vi "INI Configs FGV.vi"(6 "Config File Path":path, 7 "State":T1, 8 "error in":errorcluster, 9 "key":string, 10 "value in":string, 11 "section":string) -> (0 "error out":errorcluster, 3 "value":string)   [LabVIEW 2021]
doc: "This FGV is used to read/write config files which would contain the general configs of the application. \nBasic \"String\" config read write is implemented but it can be extended to cater to all data types."
uses:
  controls/INI FGV States.ctl
  <vilib>/Utility/config.llb/Read Key (String).vi
  <vilib>/Utility/config.llb/Write Key (String).vi
  <vilib>/Utility/config.llb/NI_LVConfig.lvlib
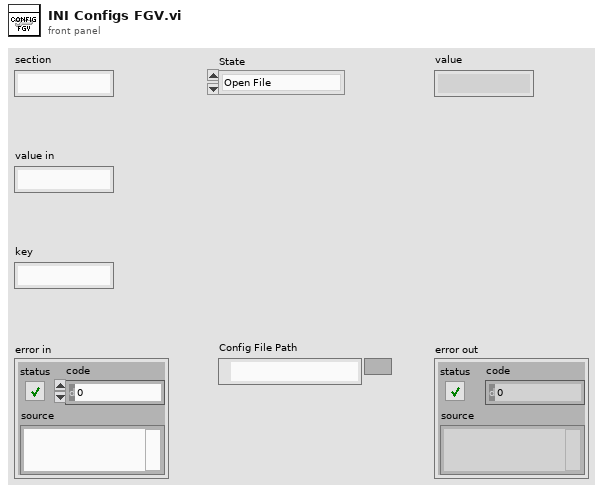
[diagram p1: front panel]
types:
  T1 = typedef "INI FGV States.ctl" = enum16{"Open File", "Read Config", "Write Config", "Close File"}
  T2 = typedef "NI_LVConfig.lvlib/Config Data RefNum.ctl" = refnum<k1>
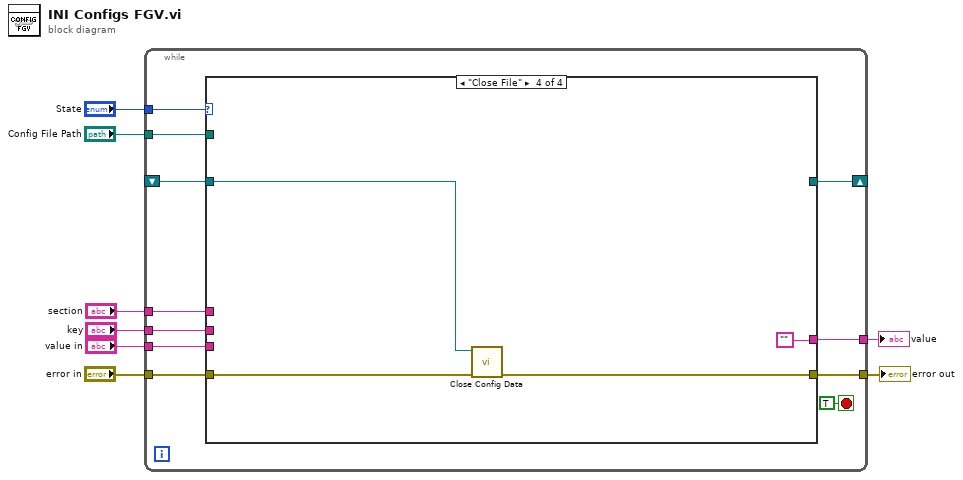
[diagram p0: block diagram]
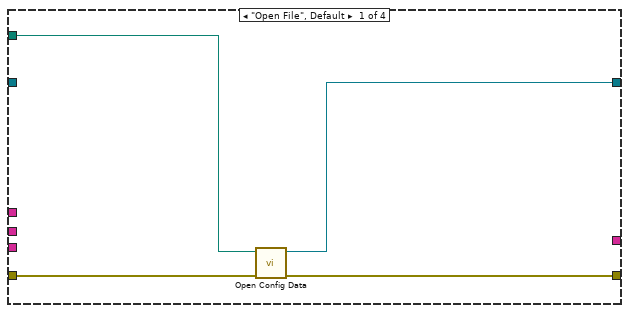
[diagram p2: hidden frame]
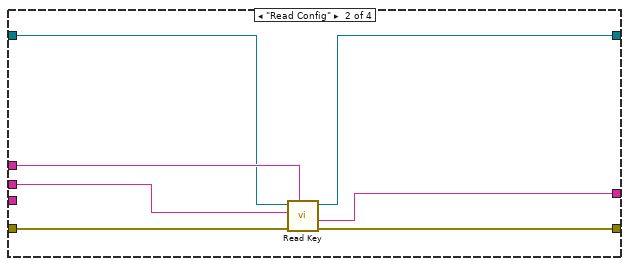
[diagram p3: hidden frame]
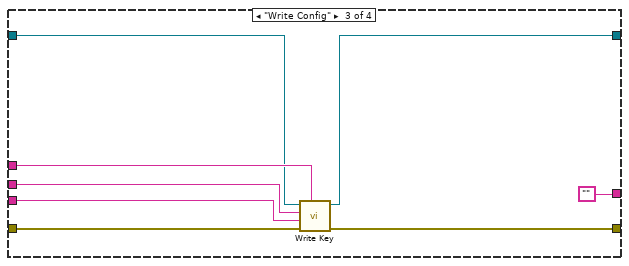
[diagram p4: hidden frame]
diagram:
  n1 = while {
    tunnel: "State" -> [w18]
    tunnel: "Config File Path" -> [w17]
    tunnel: "error in" -> [w16]
    shift-right: [w15] -> _
    shift-left: _ -> [w14]
    tunnel: [w13] -> w5
    tunnel: "section" -> [w12]
    tunnel: "key" -> [w11]
    tunnel: [w10] -> w2
    tunnel: "value in" -> [w9]
    stop <- TRUE stop-if-true
    n2 = case shown="\"Close File\"" w18 {
      tunnel: w17 -> [w23 _ _ _]
      tunnel: w16 -> [w22 w29 w37 w41]
      tunnel: [w21 w25 w31 _] -> w15
      tunnel: w14 -> [_ w26 w32 w39]
      tunnel: [w20 w29 w36 w40] -> w13
      tunnel: w12 -> [_ w28 w34 _]
      tunnel: w11 -> [_ w27 w35 _]
      tunnel: [_ w24 "" ""] -> w10
      tunnel: w9 -> [_ _ w33 _]
      frame "Open File", Default {
        n3 = call <vilib>:"Open Config Data.vi"("error in (no error)"=w22, "configuration file path"=w23) -> ("error out"=w20:errorcluster, "refnum"=w21:T2)  [unwired: 7 in, 1 out]
      }
      frame "Read Config" {
        n4 = call-poly <vilib>:"Read Key.vi"("section"=w28, "key"=w27, "refnum"=w26) -> ("value"=w24:string, "refnum out"=w25:T2)  [unwired: 5 in, 2 out]
      }
      frame "Write Config" {
        n5 = call-poly <vilib>:"Write Key.vi"("section"=w34, "error in (no error)"=w37, "value"=w33, "key"=w35, "refnum"=w32) -> ("error out"=w36:errorcluster, "refnum out"=w31:T2)  [unwired: 4 in, 1 out]
      }
      frame "Close File" {
        n6 = call <vilib>:"Close Config Data.vi"("error in (no error)"=w41, "refnum"=w39) -> ("error out"=w40:errorcluster)  [unwired: 8 in, 1 out]
      }
    }
  }
  "error out" <- w5
  "value" <- w2
